vi "PH_Beckhoff_PP_Control.start DIM Services.vi"(0 "i ref in":refnum<vi>, 5 "error in":errorcluster) -> (14 "i ref out":refnum<vi>, 19 "error out":errorcluster)   [LabVIEW 2014]
doc: "This VI starts the DIM services published by this class."
uses:
  PH_Beckhoff_PP_Control.lvlib
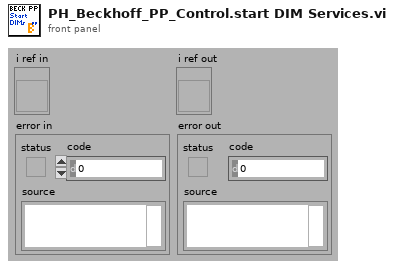
[diagram p1: front panel]
types:
  T1 = typedef "PH_Beckhoff_PP_Control.lvlib/PH_Beckhoff_PP_Control.i attribute.ctl" = cluster{"PP Conductivity Control":cluster{"PSDB":cluster{"Status Service ID":i32, "Instance ID":i32, "Data Status":T2, "Ref Status":refnum<vi>, "Error Code":i32}, "Status":cluster{"GUI Ref":refnum<vi>, "Status Service ID":i32, "Status":T3}, "DIs":cluster{"Device on":cluster{"GUI Ref":refnum<vi>, "# in Data":i32}, "Conductivity ok":cluster{"GUI Ref":refnum<vi>, "# in Data":i32}, "Temperature ok":cluster{"GUI Ref":refnum<vi>, "# in Data":i32}, "Alarm":cluster{"GUI Ref":refnum<vi>, "# in Data":i32}}, "PSDB Thread":cluster{"Ref":refnum<vi>, "Q-Ref":refnum<queue>}}, "PP Mercury Control":cluster{"PSDB":cluster{"Status Service ID":i32, "Instance ID":i32, "Data Status":T2, "Ref Status":refnum<vi>, "Error Code":i32}, "Status":cluster{"GUI Ref":refnum<vi>, "Status Service ID":i32, "Status":T3}, "on since:":cluster{"GUI Ref":refnum<vi>, "Service ID":i32, "Time":string}, "DIs":cluster{"Device on":cluster{"GUI Ref":refnum<vi>, "# in Data":i32}, "Alarm":cluster{"GUI Ref":refnum<vi>, "# in Data":i32}}, "AIs":cluster{"Concentration":cluster{"GUI Ref":refnum<vi>, "# in Data":i32}}, "PSDB Thread":cluster{"Ref":refnum<vi>, "Q-Ref":refnum<queue>}}, "PSDB":cluster{"Shot #":i32, "Subsystem":T4, "Controller":string, "Data Source":string, "Password":string}, "Handle GUI Refs Attributes":T5}
  T2 = typedef "Data_Status.ctl" = i16
  T3 = typedef "Status.ctl" = i16
  T4 = typedef "PHELIX-Subsystems.ctl" = i32
  T5 = typedef "PH Handle GUI Refs.Attributes.ctl" = cluster{"Event":refnum<user-event>, "Event registered":refnum<k4>, "GUI Refs stored":refnum<k4>}
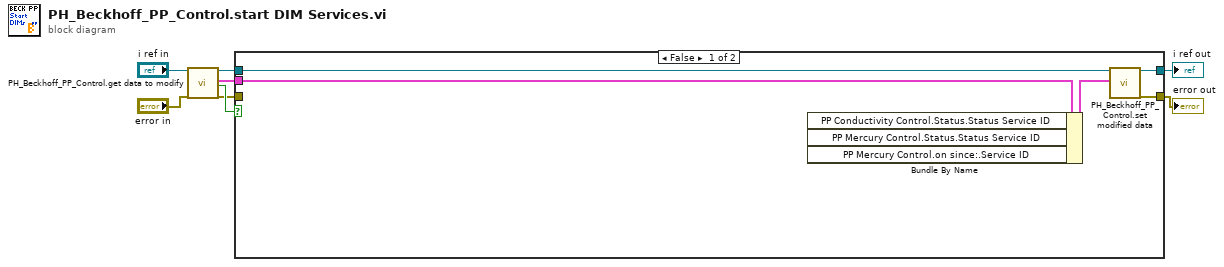
[diagram p0: block diagram]
diagram:
  n1 = call "PH_Beckhoff_PP_Control.get data to modify.vi"("i ref in"="i ref in", "error in (no error)"="error in") -> ("i ref out"=w3:refnum<vi>, "i attribute"=w1:T1, "timed out"=w4:bool, "error out"=w2:errorcluster)  [unwired: 14 in]
  n2 = case shown="False" w4 {
    tunnel: w2 -> [w13 w19]
    tunnel: [w18 w19] -> w8
    tunnel: w3 -> [w17 w20]
    tunnel: [w16 w20] -> w6
    tunnel: w1 -> [w15 _]
    frame False {
      n3 = Bundle By Name(cluster=w15) -> (w14:T1, "PP Conductivity Control.Status.Status Service ID"=w11:i32, "PP Mercury Control.Status.Status Service ID"=w10:i32, "PP Mercury Control.on since:.Service ID"=w9:i32)
      n4 = call "PH_Beckhoff_PP_Control.set modified data.vi"("i ref in"=w17, "i attribute"=w14) -> ("error in (no error)"=w12:errorcluster, "i ref out"=w16:refnum<vi>, "error out"=w18:errorcluster)  [unwired: 15 in]
    }
    frame True {
    }
  }
  "error out" <- w8
  "i ref out" <- w6
